vi "nearCamSnap.vi"(0 "采集套接字":i32, 1 "ImageData":T1, 11 "版本号":i32, 12 "error in (no error)":errorcluster) -> (4 "Image Out":T1, 8 "错误输出":string, 10 "图像统计":cluster{"mean":dbl, "variance":dbl, "最大值":u16}, 15 "error out":errorcluster)   [LabVIEW 2018]
uses:
  <vilib>/vision/Image Controls.llb/IMAQ Image.ctl
  <vilib>/vision/NI_Vision_Development_Module.lvlib
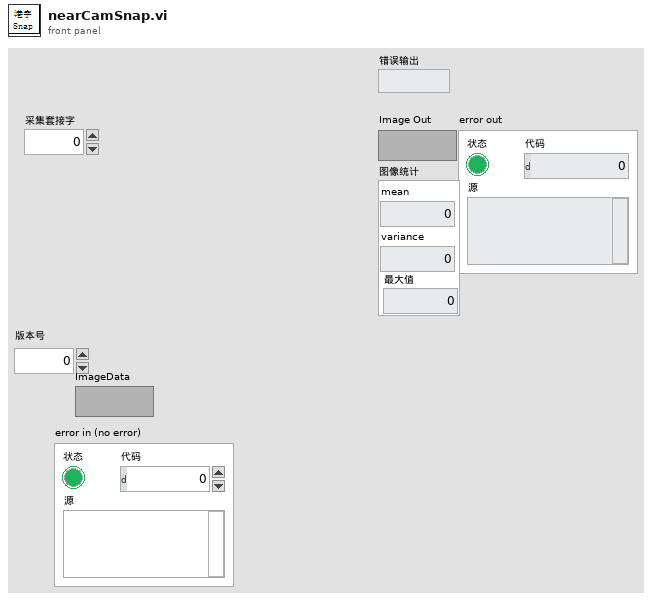
[diagram p1: front panel]
types:
  T1 = typedef "IMAQ Image.ctl" = refnum<image>
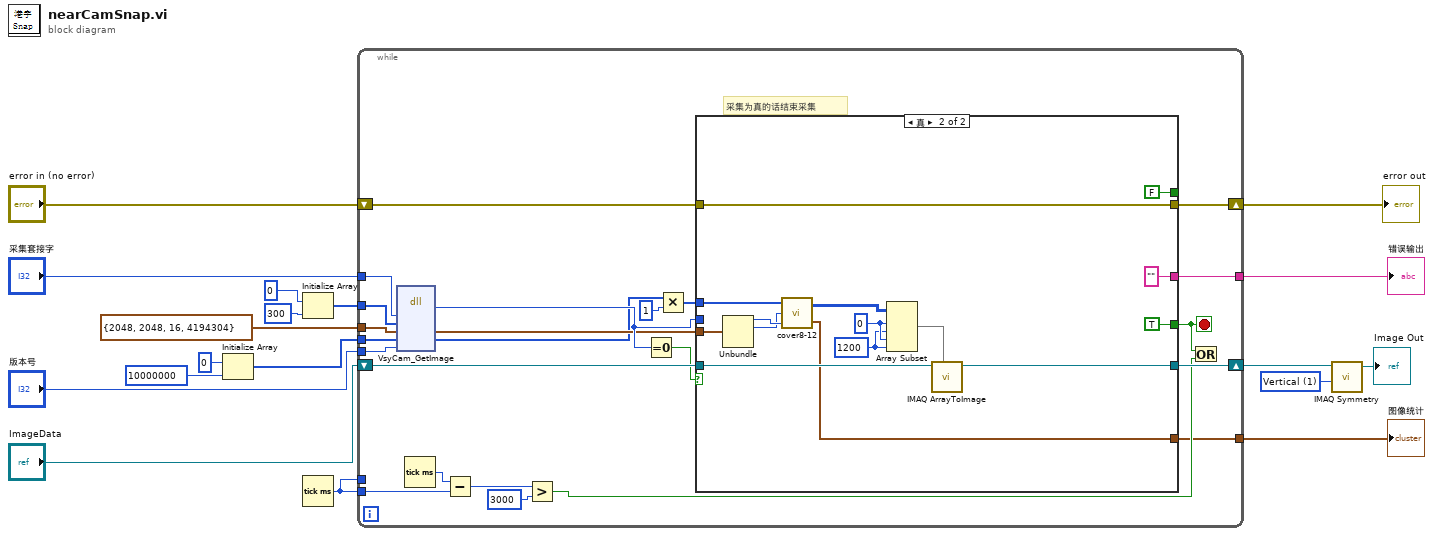
[diagram p0: block diagram]
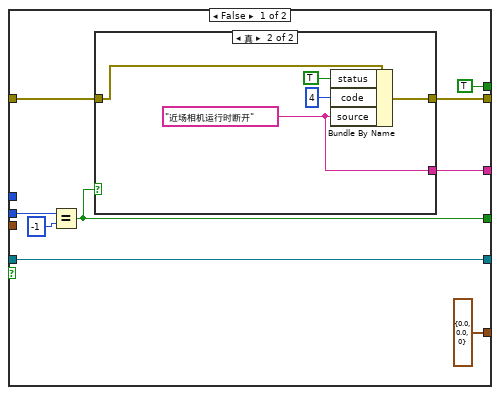
[diagram p2: hidden frame]
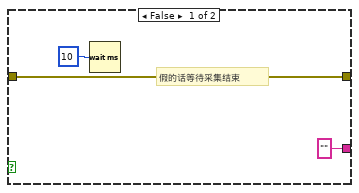
[diagram p3: hidden frame]
diagram:
  w1 = u32 1 items=["Horizontal", "Vertical", "Central", "1st Diagonal", "2nd Diagonal"] ("Type of Symmetry")
  n1 = Initialize Array(u8 0 ("元素"), 10000000) -> (w4:u8[])
  n2 = Initialize Array(u8 0, 300) -> (w8:u8[])
  n3 = Tick Count (ms)() -> (millisecond timer value=w14:u32)
  n4 = while {
    shift-right: [w38] -> w16
    shift-left: "error in (no error)" -> [w41]
    shift-right: [w39] -> w3
    shift-left: "ImageData" -> [w40]
    tunnel: [w37] -> w15
    tunnel: w14 -> [_]
    tunnel: w14 -> [w32]
    tunnel: "采集套接字" -> [w30]
    tunnel: w8 -> [w29]
    tunnel: cluster{i32, i32, i32, i32} {2048, 2048, 16, 4194304} ("簇") -> [w28]
    tunnel: w4 -> [w27]
    tunnel: "版本号" -> [w26]
    tunnel: [w22] -> w11
    stop <- w31 stop-if-true
    # "采集为真的话结束采集"
    n5 = dll-call lib="PTH2^abs E航天测量驱动相机驱动LabView2014Demo_V1.0.8\nLabView14Demo\nVsyCam.dll" fn="VsyCam_GetImage" label="VsyCam_GetImageVsyCam_GetImage"("sockFd"=w30, "Header"=w29, w28, "Data"=w27, "version"=w26) -> ("返回类型"=w24:i32, w23:cluster{i32, i32, i32, i32}, "Data"=w21:u8[])  [unwired: 6 in, 2 out]
    n6 = Tick Count (ms)() -> (millisecond timer value=w36:u32)
    n7 = Subtract(x=w36, y=w32) -> (x-y=w35:u32)
    n8 = Greater?(x=w35, y=u32 3000) -> (0:w33:bool)
    n9 = Equal To 0?(x=w24) -> (x = 0?=w25:bool)
    n10 = Multiply(x=w21, y=1) -> (x*y=w19:i32[])
    n11 = case shown="真" w25 {
      tunnel: w23 -> [_ w73]
      tunnel: w19 -> [_ w72]
      tunnel: w40 -> [w44 w69]
      tunnel: w41 -> [w47 w67]
      tunnel: [w50 w67] -> w38
      tunnel: [TRUE FALSE] -> _
      tunnel: [w48 "" ("source")] -> w37
      tunnel: w24 -> [w46 _]
      tunnel: [w44 w65] -> w39
      tunnel: [w43 TRUE] -> w31
      tunnel: [cluster{"mean":dbl, "variance":dbl, "最大值":u16} {"mean"=0.0, "variance"=0.0, "最大值"=0} ("统计输出") w63] -> w22
      frame False {
        n12 = Equal?(x=w46, y=-1) -> (x = y?=w43:bool)
        n13 = case shown="真" w43 {
          tunnel: [w53 w56] -> w50
          tunnel: ["" ("source") w55] -> w48
          tunnel: w47 -> [w53 w54]
          frame False {
            # "假的话等待采集结束"
            n14 = Wait (ms)(milliseconds to wait=u32 10 ("等待时间（毫秒）")) -> ()  [unwired: 1 out]
          }
          frame True {
            w55 = "近场相机运行时断开" ("source")
            n15 = Bundle By Name(cluster=w54, "status"=TRUE, "code"=4, "source"=w55) -> (w56:errorcluster)
          }
        }
      }
      frame True {
        w60 = 1200 ("长度")
        w61 = 0 ("索引")
        n16 = Unbundle(w73) -> (w71:i32, w70:i32)  [unwired: 2 out]
        n17 = call "cover8-12.vi"("H"=w71, "W"=w70, "Image Data"=w72) -> ("统计输出"=w63:cluster{"mean":dbl, "variance":dbl, "最大值":u16}, "PIC Out"=w62:u16[][])
        n18 = Array Subset(array=w62, index (row)=w61, length (row)=w60, index (col)=w61, length (col)=w60) -> (w59:u16[][])
        n19 = call "IMAQ ArrayToImage"("Image Pixels (U16)"=w59, "Image"=w69) -> ("Image Out"=w65:T1)  [unwired: 8 in, 1 out]
      }
    }
    n20 = Or(x=w31, y=w33) -> ()  [unwired: 1 out]
  }
  "error out" <- w16
  "错误输出" <- w15
  "图像统计" <- w11
  n21 = call "IMAQ Symmetry"("Type of Symmetry"=w1, "Image Src"=w3) -> ("Image Dst Out"=→"Image Out":T1)  [unwired: 3 in, 1 out]
